vi "Write_RobotLiftOutput.vi"(8 "error in (no error)":errorcluster, 10 "RobotLiftOutput":T1, 11 "RobotLiftData in":refnum<class "RobotLiftData.lvclass">) -> (0 "error out":errorcluster, 3 "RobotLiftData out":refnum<class "RobotLiftData.lvclass">)   [LabVIEW 2017, in "RobotLiftData.lvclass"]
uses:
  RobotLiftData.lvclass
  Team-code/RobotLiftOutput.ctl
  RobotLiftData.lvclass/RobotLiftData.ctl
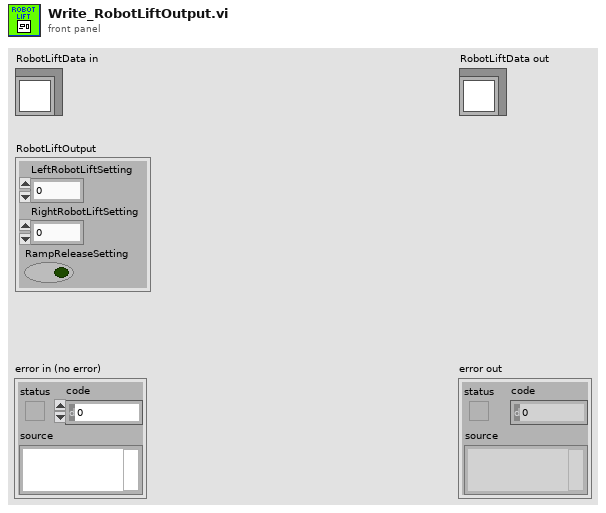
[diagram p1: front panel]
types:
  T1 = typedef "RobotLiftData.lvclass/RobotLiftOutput.ctl" = cluster{"LeftRobotLiftSetting":dbl, "RightRobotLiftSetting":dbl, "RampReleaseSetting":bool}
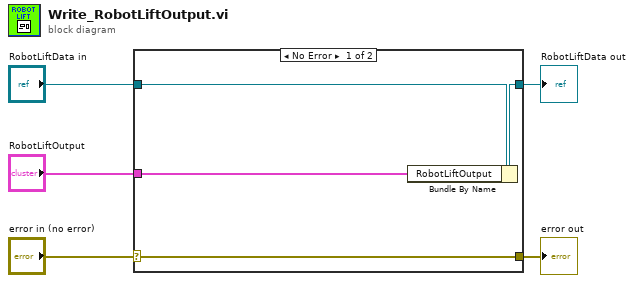
[diagram p0: block diagram]
diagram:
  n1 = case shown="No Error" "error in (no error)" {
    selector: "error in (no error)" -> [w9 w10]
    tunnel: [w9 w10] -> w4
    tunnel: [w7 w11] -> w2
    tunnel: "RobotLiftData in" -> [w8 w11]
    tunnel: "RobotLiftOutput" -> [w6 _]
    frame No Error {
      n2 = Bundle By Name(cluster=w8, "RobotLiftOutput"=w6) -> (w7:refnum<class "RobotLiftData.lvclass">)
    }
    frame Error {
    }
  }
  "error out" <- w4
  "RobotLiftData out" <- w2
